vi "Save Chunk.vi"(4 "Volatge Y":dbl[](array[numeric]), 8 "error in (no error)":errorcluster, 9 "Voltage X":dbl[](array[numeric]), 10 "Frequency":dbl[](array[numeric]), 11 "Spectrum Recorder in":refnum<class "Spectrum Recorder too.lvclass">) -> (0 "error out":errorcluster, 3 "Spectrum Recorder out":refnum<class "Spectrum Recorder too.lvclass">)   [LabVIEW 2016, in "Spectrum Recorder too.lvclass"]
uses:
  Spectrum Recorder too.lvclass
  C:/github/LabActor/Template Module/Template Module.lvclass
  C:/Program Files/National Instruments/LabVIEW 2016/vi.lib/ActorFramework/Actor/Actor.lvclass
  Template Module/Template Module.lvclass/Template Module.ctl
  <vilib>/ActorFramework/Actor/Actor.lvclass/Actor.ctl
  Spectrum Recorder too.lvclass/Spectrum Recorder too.ctl
  Controllers/Process Controller Messages/Update Plots Msg/Update Plots Msg.lvclass/Update Plots Msg.ctl
  <vilib>/ActorFramework/Message Enqueuer/Message Enqueuer.lvclass/Message Enqueuer.ctl
  Template Module/Read Logger.vi
  <vilib>/ActorFramework/Message Enqueuer/Enqueue.vi
  Controllers/Process Controller Messages/Update Plots Msg/Update Plots Msg.lvclass
  C:/Program Files/National Instruments/LabVIEW 2016/vi.lib/ActorFramework/Message/Message.lvclass
  <vilib>/ActorFramework/Message Priority Queue/Priority Enqueue.vi
  Loggers/Logger/Logger.lvclass
  <vilib>/ActorFramework/Actor/Actor.lvclass
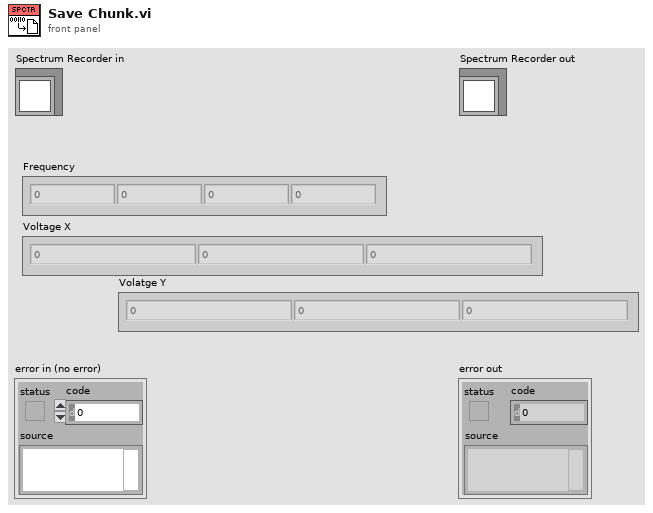
[diagram p1: front panel]
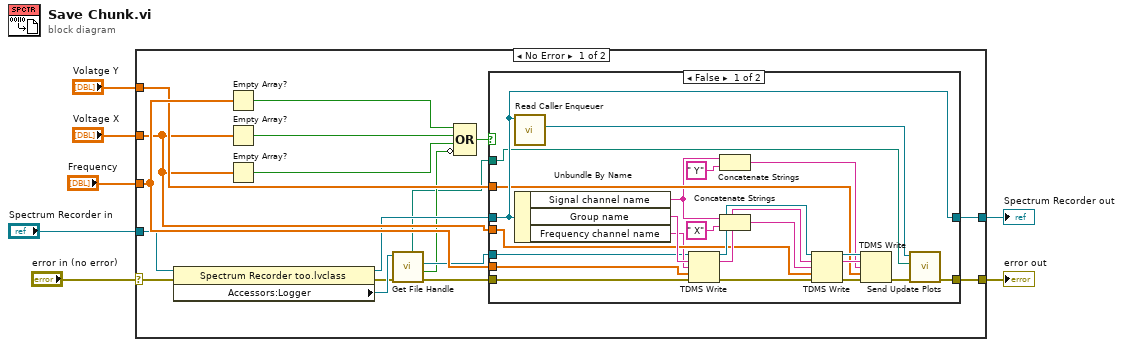
[diagram p0: block diagram]
diagram:
  n1 = case shown="No Error" "error in (no error)" {
    selector: "error in (no error)" -> [w24 w52]
    tunnel: [w23 w52] -> w6
    tunnel: [w25 w51] -> w4
    tunnel: "Spectrum Recorder in" -> [w15 w51]
    tunnel: "Voltage X" -> [w17 _]
    tunnel: "Frequency" -> [w19 _]
    tunnel: "Volatge Y" -> [w18 _]
    frame No Error {
      n2 = property class="Spectrum Recorder too.lvclass"(reference=w15, error in=w24) -> (reference out=w14:refnum<class "Spectrum Recorder too.lvclass">, error out=w12:errorcluster, "Accessors:Logger"=w13:refnum<class "Logger.lvclass">)
      n3 = Empty Array?(array=w19) -> (empty?=w22:bool)
      n4 = Empty Array?(array=w17) -> (empty?=w21:bool)
      n5 = Empty Array?(array=w17) -> (empty?=w16:bool)
      n6 = call-dynamic "Get File Handle.vi"("error in (no error)"=w12, "Logger in"=w13) -> ("error out"=w11:errorcluster, "Valid"=w9:bool, "File handle"=w10:refnum<k34>, "Data File  Path"=w8:path)  [unwired: 5 in, 1 out]
      n7 = Compound Arithmetic op=OR(w22, w21, w16, invert w9) -> (w20:bool)
      n8 = case shown="False" w20 {
        tunnel: w17 -> [w42 _]
        tunnel: w19 -> [w46 _]
        tunnel: w14 -> [w40 w50]
        tunnel: [w40 w50] -> w25
        tunnel: w11 -> [w47 w49]
        tunnel: [w29 w49] -> w23
        tunnel: w18 -> [w36 _]
        tunnel: w10 -> [w27 _]
        tunnel: w8 -> [w26 _]
        frame False {
          n9 = call <vilib>:"Read Caller Enqueuer.vi"("Actor"=w40) -> ("Caller Enqueuer"=w30:refnum<class "Message Enqueuer.lvclass">)  [unwired: 10 in]
          n10 = Unbundle By Name(w40) -> ("Signal channel name"=w31:string, "Group name"=w48:string, "Frequency channel name"=w41:string)
          n11 = TDMS Write(0:w27, 5:w48, 7:w41, 9:w46, 11:w47) -> (4:w44:refnum<k34>, 6:w43:string, 15:w45:errorcluster)  [unwired: 1 in, 1 out]
          n12 = Concatenate Strings(w31, " Y" ("string")) -> (w32:string)
          n13 = Concatenate Strings(w31, " X" ("string")) -> (w34:string)
          n14 = TDMS Write(0:w44, 5:w43, 7:w34, 9:w42, 11:w45) -> (4:w38:refnum<k34>, 6:w37:string, 15:w39:errorcluster)  [unwired: 1 in, 1 out]
          n15 = TDMS Write(0:w38, 5:w37, 7:w32, 9:w36, 11:w39) -> (15:w28:errorcluster)  [unwired: 1 in, 3 out]
          n16 = call "Send Update Plots.vi"("error in (no error)"=w28, "File Path"=w26, "Message Enqueuer"=w30) -> ("error out"=w29:errorcluster)  [unwired: 7 in, 1 out]
        }
        frame True {
        }
      }
    }
    frame Error {
    }
  }
  "error out" <- w6
  "Spectrum Recorder out" <- w4
